vi "Alt C.vi"(0 "FrontLeg PS":bool=TRUE, 1 "Old State":string, 2 "BackLeg PS":bool=TRUE, 4 "MidLeg Up":bool=TRUE, 5 "BackLeg Up":bool=TRUE, 6 "MidLeg PS":bool=TRUE, 8 "Front Leg Up":bool, 9 "Back Claws Cmd":bool=TRUE, 11 "Front Claw Cmd":bool=TRUE) -> (13 "Drive Motor Enabled":bool=TRUE, 14 "Mid Leg Comd":enum16{"Down Closed", "Down Opened", "Up"}(ring), 15 "New State":string, 16 "Front Leg Cmd":enum16{"Down Closed", "Down Opened", "Up"}(ring), 17 "Skids":bool, 18 "Engage Back Leg":bool)   [LabVIEW 2012]
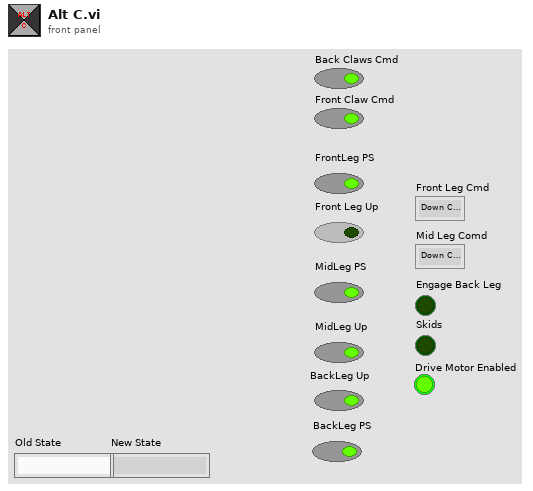
[diagram p1: front panel]
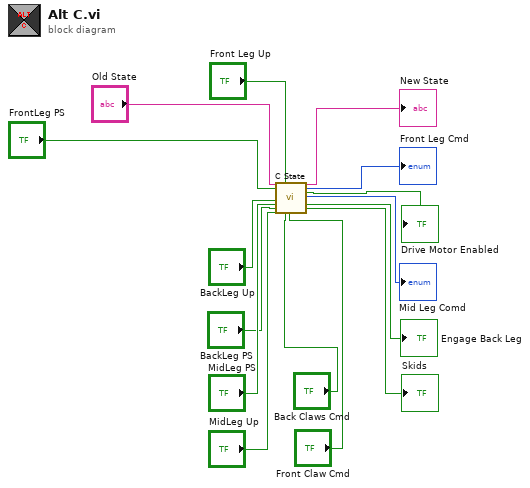
[diagram p0: block diagram]
diagram:
  n1 = call "C State.vi"("State"="Old State", "Front Leg PS"="FrontLeg PS", "Back Leg Up"="BackLeg Up", "Mid Leg PS"="MidLeg PS", "Back Leg PS"="BackLeg PS", "Mid Leg Up"="MidLeg Up", "Front Leg Up"="Front Leg Up", "Back Claws Cmd"="Back Claws Cmd", "Front Claw Cmd"="Front Claw Cmd") -> ("newState"=→"New State":string, "Front Leg Cmd"=→"Front Leg Cmd":enum16{"Down Closed", "Down Opened", "Up"}, "Drive Motor Enabled"=→"Drive Motor Enabled":bool, "Mid Leg Cmd"=→"Mid Leg Comd":enum16{"Down Closed", "Down Opened", "Up"}, "Engage Back Leg"=→"Engage Back Leg":bool, "Skids"=→"Skids":bool)  [unwired: 13 in]
